vi "qSPV.vi"(0 "System no.":i32=1 min=1 max=4 step=1, 1 "Target Memory Type":T1, 2 "ContainerUnit":string, 3 "FunctionUnit":string, 4 "ParameterID":string, 5 "error in":errorcluster) -> (14 "Values":string[](array[string]), 19 "error out":errorcluster)   [LabVIEW 2026]
doc: "SPV? (Get Parameter Value)\n\nDescription\nReads parameter values from the memories of the controller.\nDepending on the argument(s) used, the query is limited to a certain memory type and certain \nparameters.\n\nFormat\nSPV?[ <MemType>[ <Container Unit>[ <Function Unit>[ <ParameterID>]]]]\n\nArguments\nSPV? without arguments queries the values of all parameters that can be read in the current \nuser command level (p. 69) in all memories. \nThe available parameters and their properties (including <Container Unit>, <Function Unit>, \n<ParameterID>, dimension of the parameter, data type and range for the parameter value) can \nbe queried with the USG? PAM command (p. 77). \n<MemType>\nType of memory from which the values are to be read\nIf no further arguments are specified, all parameters are queried from the specified memory.\nIf the placeholder \"*\" is specified for <MemType>, all memories are queried.\nPossible values:\nRAM, TMP, FLASH\n* as placeholder\n<Container Unit>\nContainer unit, whose parameters are to be queriedIf only the <MemType> and <Container \nUnit> arguments are specified, all parameters of the container unit and the function units it \ncontains in the specified memory are queried.\nPossible values: Alias of the container unit (p. 94) \n<Function Unit>\nFunction unit, whose parameters are to be queriedIf only the <MemType>, <Container Unit> \nand <Function Unit> arguments are specified, all parameters of the function unit are queried in\nthe specified memory.\nIf only the parameters that belong directly to the <Container Unit> are to be queried, \"-\" must \nbe entered for <Function Unit>.\nPossible values:\nAlias of the function unit (p. 94) \n\"-\" \n<ParameterID>\nThe value of the parameter addressed by <Container Unit>, <Function Unit> and <ParameterID> \nwill be queried in the specified memory.\n<ParameterID> always contains a parameter identifier in hexadecimal format. For 0-\ndimensional parameters, <ParameterID> is fully specified by the parameter identifier.\nFor one-dimensional and multi-dimensional parameters, an element address is also required \ntogether with the parameter identifier. Depending on the dimension of the parameter, the \nelement address consists of one or more parts that are separated from the parameter identifier \nand each other by a comma.\n- One-dimensional parameter (vector) ? the element address is ,number\n- Two-dimensional parameter (two-dimensional matrix) ? the element address is \n,number,number\n- Three-dimensional parameter (three-dimensional matrix) ? the element address \nis ,number,number,number\nThe address data for the parameters can be queried with USG? PAM (p. 77). \nPossible values:\n0x0000 to 0xFFFF\nFor one-dimensional and multi-dimensional parameters, an additional integer = 1 for each \ndimension\n\nResponse\n{<MemType> <Container Unit> <Function Unit> <ParameterID>\"=\"<Value> LF}\n\nNotes\nThe response to USG? PAM includes amongst other things the user command level for the read \naccess (<READ-UCL> column) to the parameter value. The UCL? command (p. 71) queries the \nactive user command level. Use the UCL command (p. 69) to change to the appropriate user \ncommand level.\nThe value of a Configuration parameter can be set in the different memories of the controller \nusing the SPV command (p. 60). \nThe CPA command (p. 8) can be used to copy the values of configuration parameters between \nthe different memories of the controller.\nIf the flash memory is queried with the command SPV?, the <Value> for \"Configuration\" \nparameters will be \"-\" if values have not been saved to the flash memory for these parameters \n(e.g. using SPV or CPA).\nFor further details, see \"Parameter Handling - GCS 3.0\" (p. 119). \n\nUser command level\nUSR"
uses:
  ConfigurationMemoryType.ctl
  <vilib>/Utility/error.llb/Trim Whitespace One-Sided.vi
panel:
  # "SPV? (Get Parameter Value)\n\nReads parameter values from the memories of the controller.\nDepending on the argument(s) used, the query is limited to a certain memory type and certain \nparameters."
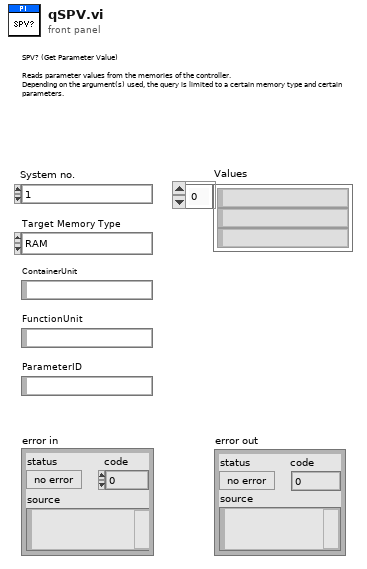
[diagram p1: front panel]
types:
  T1 = typedef "ConfigurationMemoryType.ctl" = enum16{"RAM", "TMP", "FLASH"}
  T2 = typedef "Syntax.ctl" = enum16{"GCS 1.0", "GCS 2.0", "GCS 3.0"}
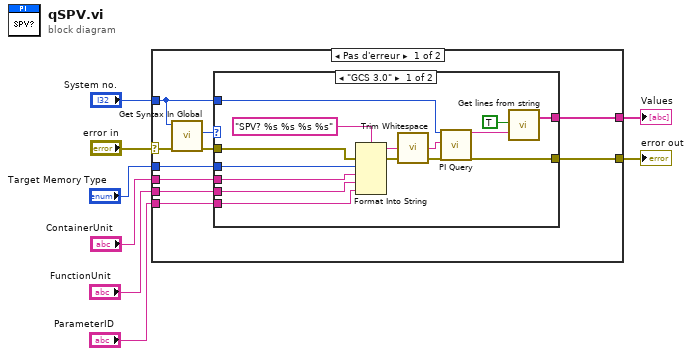
[diagram p0: block diagram]
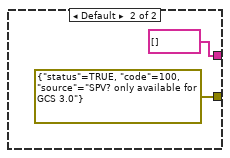
[diagram p2: hidden frame]
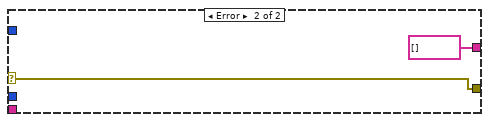
[diagram p3: hidden frame]
diagram:
  n1 = case shown="Pas d'erreur" "error in" {
    selector: "error in" -> [w16 w36]
    tunnel: [w15 w36] -> w7
    tunnel: [w9 string[] [] ("Values")] -> w6
    tunnel: "System no." -> [w10 _]
    tunnel: "Target Memory Type" -> [w14 _]
    tunnel: "ContainerUnit" -> [w13 _]
    tunnel: "FunctionUnit" -> [w12 _]
    tunnel: "ParameterID" -> [w11 _]
    frame No Error {
      n2 = call "Get Syntax In Global.vi"("error in"=w16, "System no."=w10) -> ("error out"=w18:errorcluster, "Syntax"=w17:T2)  [unwired: 8 in]
      n3 = case shown="\"GCS 3.0\"" w17 {
        tunnel: [w20 errorcluster {"status"=TRUE, "code"=100, "source"="SPV? only available for GCS 3.0"} ("error out")] -> w15
        tunnel: w18 -> [w30 _]
        tunnel: w10 -> [w24 _]
        tunnel: w14 -> [w29 _]
        tunnel: w13 -> [w28 _]
        tunnel: w12 -> [w27 _]
        tunnel: w11 -> [w26 _]
        tunnel: [w21 string[] [] ("Values")] -> w9
        frame "GCS 3.0" {
          n4 = Format Into String(format string="SPV? %s %s %s %s", error in=w30, w29, w28, w27, w26) -> (resulting string=w32:string, error out=w25:errorcluster)  [unwired: 1 in]
          n5 = call <vilib>:"Trim Whitespace.vi"("string"=w32) -> ("trimmed string"=w23:string)  [unwired: 1 in]
          n6 = call "PI Query.vi"("System no."=w24, "String to send"=w23, "error in"=w25) -> ("String read"=w19:string, "error out"=w20:errorcluster)  [unwired: 13 in, 2 out]
          n7 = call "Get lines from string.vi"("Cut spaces?"=TRUE, "Input string"=w19) -> ("Strings"=w21:string[])  [unwired: 16 in, 1 out]
        }
        frame Default {
        }
      }
    }
    frame Error {
    }
  }
  "error out" <- w7
  "Values" <- w6
